vi "Status SpecimenTempCtrlSettings(P).vi"(8 "error in (no error)":errorcluster, 10 "Address (0)":i32, 11 "VISA resource name":refnum<visa-resource-name>) -> (0 "error out":errorcluster, 2 "control permission/state":bool, 3 "VISA resource name out":refnum<visa-resource-name>, 4 "lower deviation":dbl, 5 "upper deviation":dbl)   [LabVIEW 2016, in "Environment Chamber.lvlib" / "Climatic Chamber.lvlib"]
doc: "<b>Operating specimen temperature control monitor</B>\n\nReturns the specimen temperature control state."
uses:
  Climatic Chamber.lvlib
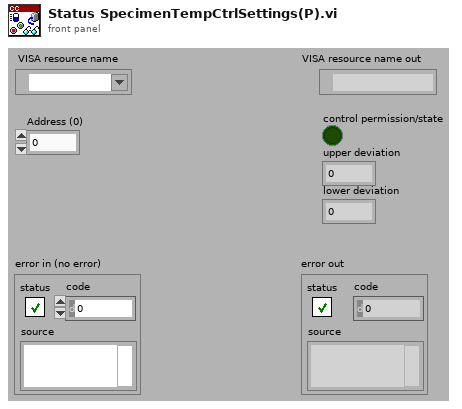
[diagram p1: front panel]
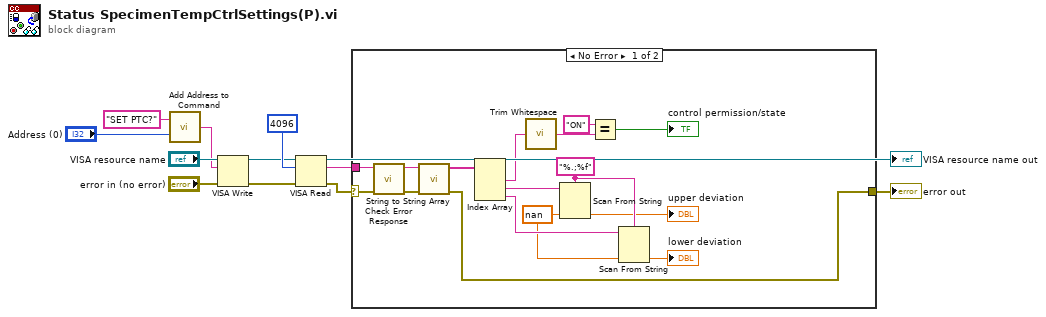
[diagram p0: block diagram]
diagram:
  n1 = call "Add Address to Command.vi"("Address (0)"="Address (0)", "Command"="SET PTC?") -> ("Command OUT"=w5:string)
  n2 = VISA Write(VISA resource name="VISA resource name", write buffer=w5, error in (no error)="error in (no error)") -> (VISA resource name out=w9:refnum<visa-resource-name>, error out=w8:errorcluster)  [unwired: 1 out]
  n3 = VISA Read(VISA resource name=w9, byte count=u32 4096, error in (no error)=w8) -> (VISA resource name out=→"VISA resource name out":refnum<visa-resource-name>, read buffer=w3:string, error out=w4:errorcluster)  [unwired: 1 out]
  n4 = case shown="No Error" w4 {
    selector: w4 -> [w27 w29]
    tunnel: w3 -> [w28 _]
    tunnel: [w16 w29] -> w2
    frame No Error {
      w17 = nan ("default value 1")
      w18 = "%.;%f" ("format string")
      n5 = call "Check Error Response.vi"("error in (no error)"=w27, "read String"=w28) -> ("error out"=w26:errorcluster, "String out"=w25:string)  [unwired: 7 in, 1 out]
      n6 = call "String to String Array.vi"("error in (no error)"=w26, "String received"=w25) -> ("error out"=w16:errorcluster, "Array Data"=w24:string[])  [unwired: 8 in]
      n7 = Index Array(array=w24) -> (element #1=w23:string, element #2=w20:string, element #3=w19:string)  [unwired: 3 in]
      n8 = call <vilib>:"Trim Whitespace.vi"("string"=w23) -> ("trimmed string"=w22:string)  [unwired: 1 in]
      n9 = Scan From String(format string=w18, input string=w20, default 1=w17) -> (output 1=→"upper deviation":dbl)  [unwired: 2 in, 3 out]
      n10 = Equal?(x="ON", y=w22) -> (x = y?=→"control permission/state":bool)
      n11 = Scan From String(format string=w18, input string=w19, default 1=w17) -> (output 1=→"lower deviation":dbl)  [unwired: 2 in, 3 out]
    }
    frame Error {
    }
  }
  "error out" <- w2
